vi "SetCryo.vi"(8 "error in (no error)":errorcluster, 9 "Head":bool, 10 "System":bool, 11 "PTC10":refnum<visa-resource-name>) -> (0 "error out":errorcluster)   [LabVIEW 2023]
uses:
  <instrlib>/Stanford PTC10/SRS PTC10.lvlib
panel:
  out "SRS PTC10 VISA out":refnum<visa-resource-name>
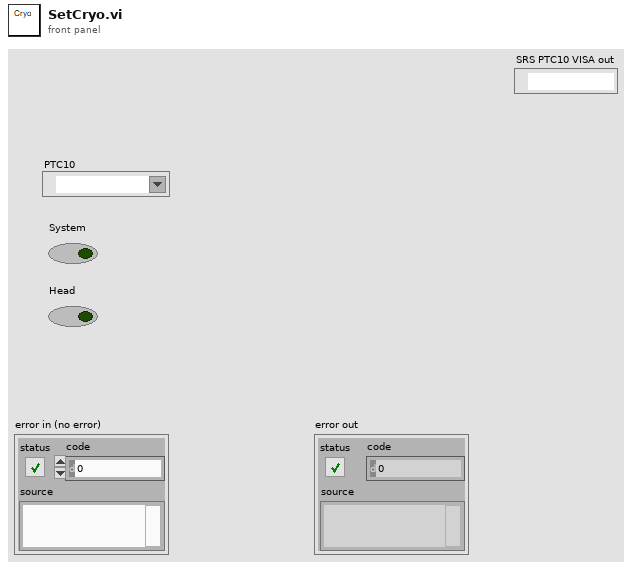
[diagram p1: front panel]
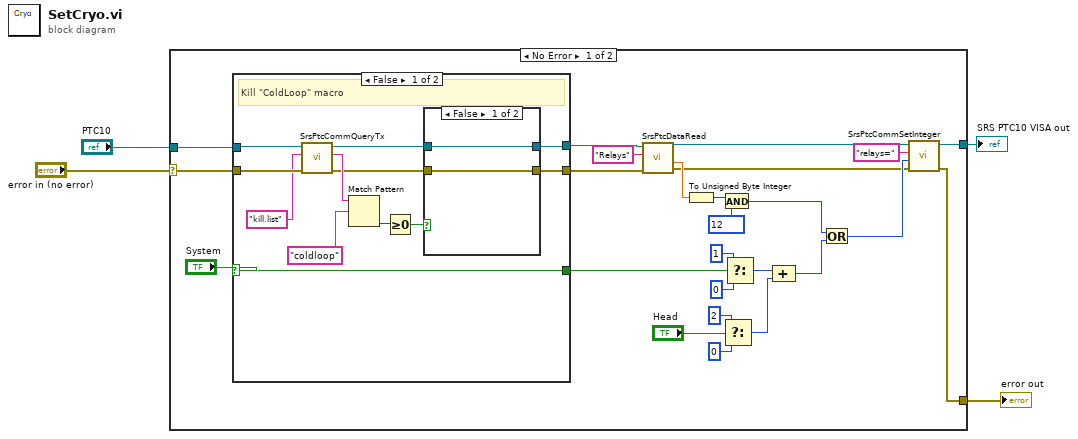
[diagram p0: block diagram]
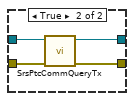
[diagram p2: hidden frame]
diagram:
  n1 = case shown="No Error" "error in (no error)" {
    selector: "error in (no error)" -> [w6 w52]
    tunnel: "PTC10" -> [w8 w51]
    tunnel: [w12 w52] -> w2
    tunnel: [w11 w51] -> w1
    frame No Error {
      n2 = case shown="False" "System" {
        selector: "System" -> [w41 w50]
        tunnel: [w41 w50] -> w9
        tunnel: w8 -> [w40 w49]
        tunnel: [w30 w49] -> w7
        tunnel: w6 -> [w39 w48]
        tunnel: [w31 w48] -> w5
        frame False {
          # "Kill \"ColdLoop\" macro"
          n3 = call <instrlib>:"SrsPtcCommQueryTx.vi"("error in"=w39, "Query"="kill.list", "SRS PTC10 VISA in"=w40) -> ("error out"=w32:errorcluster, "Query sent"=w37:string, "SRS PTC10 VISA out"=w33:refnum<visa-resource-name>)  [unwired: 6 in]
          n4 = Match Pattern(string=w37, regular expression="coldloop") -> (offset past match=w35:i32)  [unwired: 1 in, 3 out]
          n5 = Greater Or Equal To 0?(x=w35) -> (x >= 0?=w34:bool)
          n6 = case shown="False" w34 {
            tunnel: w33 -> [w43 w47]
            tunnel: w32 -> [w42 w46]
            tunnel: [w42 w45] -> w31
            tunnel: [w43 w44] -> w30
            frame False {
            }
            frame True {
              n7 = call <instrlib>:"SrsPtcCommQueryTx.vi"("error in"=w46, "SRS PTC10 VISA in"=w47) -> ("error out"=w45:errorcluster, "SRS PTC10 VISA out"=w44:refnum<visa-resource-name>)  [unwired: 7 in, 1 out]
            }
          }
        }
        frame True {
        }
      }
      n8 = call <instrlib>:"SrsPtcDataRead.vi"("error in"=w5, "Channel"="Relays", "SRS PTC10 VISA in"=w7) -> ("error out"=w13:errorcluster, "Output as number"=w28:dbl, "SRS PTC10 VISA out"=w14:refnum<visa-resource-name>)  [unwired: 5 in, 1 out]
      n9 = To Unsigned Byte Integer(number=w28) -> (unsigned 8bit integer=w27:u8)
      n10 = And(x=w27, y=u8 12) -> (x .and. y?=w18:u8)
      n11 = Select(t=u8 2, s="Head", f=u8 0) -> (s? t:f=w19:u8)
      n12 = Select(t=u8 1, s=w9, f=u8 0) -> (s? t:f=w20:u8)
      n13 = Compound Arithmetic op=ADD(w20, w19) -> (w17:u8)
      n14 = Or(x=w18, y=w17) -> (x .or. y?=w16:u8)
      n15 = call <instrlib>:"SrsPtcCommSetInteger.vi"("error in"=w13, "Value"=w16, "Command"="relays=", "SRS PTC10 VISA in"=w14) -> ("error out"=w12:errorcluster, "SRS PTC10 VISA out"=w11:refnum<visa-resource-name>)  [unwired: 2 out]
    }
    frame Error {
    }
  }
  "error out" <- w2
  "SRS PTC10 VISA out" <- w1
